vi "Autonomous Independent.vi"   [LabVIEW 2013]
doc: "This VI is called when autonomous begins, and will automatically be terminated when autonomous ends. You can carry out timed or sensor driven robot movement independently without needing to return to the caller."
uses:
  <vilib>/Rock Robotics/WPI/Solenoid/WPI_SolenoidValue.ctl
  Robot Global Data.vi
  <vilib>/Rock Robotics/WPI/RobotDrive/WPI_RobotDriveGetSetRefNum.vi
  <vilib>/Rock Robotics/WPI/Solenoid/WPI_SolenoidSetEnum.vi
  <vilib>/Rock Robotics/WPI/Joystick/WPI_JoystickGetSetRefNum.vi
panel:
  # "Be sure to right-click and choose Data Operations>>Make Current Value default if you want to save the array values with the VI"
types:
  T1 = typedef "WPI_JoystickDevRef.ctl" = cluster{"Device":T2}
  T2 = typedef "WPI_JoystickDeviceEnum.ctl" = enum16{"USB 1", "USB 2", "USB 3", "USB 4", "Kinect 1", "Kinect 2"}
  T3 = cluster{"axis 1 (x)":dbl, "axis 2 (y)":dbl, "axis 3 (throttle)":dbl, "axis 4":dbl, "axis 5":dbl, "axis 6":dbl}
  T4 = typedef "WPI_RobotDriveDevRef.ctl" = cluster{"DevStatus":errorcluster, "Motors[]":T5[], "Square Inputs":bool, "Max Output":dbl, "Isochronous":bool}
  T5 = typedef "WPI_MotorControlDeviceRef.ctl" = cluster{"DeviceStatus":errorcluster, "Type":enum16{"PWM", "CAN"}, "PWM":cluster{"Digital Module":T6, "PWM Channel":T7, "DeadBand":T8}, "CAN":cluster{"Device Number":u8, "Control Mode":T9, "Semaphore":T10, "Max Vout":dbl}, "Invert":bool, "TransformRef":T11, "InvTransformRef":T11}
  T6 = typedef "FPGA_TypedefDigitalModule.ctl" = enum16{"Digital Module 1", "Digital Module 2"}
  T7 = typedef "FPGA_DIOPWMChannel.ctl" = enum8{"PWM 1", "PWM 2", "PWM 3", "PWM 4", "PWM 5", "PWM 6", "PWM 7", "PWM 8", "PWM 9", "PWM 10", "Invalid"}
  T8 = typedef "WPI_PWMDeadband.ctl" = cluster{"Name":string, "maxPositivePwm":i32, "minPositivePwm":i32, "centerPwm":i32, "maxNegativePwm":i32, "minNegativePwm":i32, "angularRange":u16}
  T9 = typedef "WPI_CANJaguar_ControlMode.ctl" = enum8{"Percent VBus", "Current", "Speed", "Position", "Voltage"}
  T10 = typedef "Semaphore RefNum" = refnum<k1>
  T11 = typedef "WPI_PWMTransform_ConPane.ctl" = refnum<vi>
  T12 = typedef "WPI_SolenoidDevRef.ctl" = cluster{"DevStatus":errorcluster, "Solenoid Module":T13, "Forward Solenoid Channel":T14, "Reverse Solenoid Channel":T14}
  T13 = typedef "FPGA_TypedefSolenoidModule.ctl" = enum16{"Solenoid Module 1", "Solenoid Module 2"}
  T14 = typedef "WPI_SolenoidChannel.ctl" = enum8{"Solenoid 1", "Solenoid 2", "Solenoid 3", "Solenoid 4", "Solenoid 5", "Solenoid 6", "Solenoid 7", "Solenoid 8", "Invalid"}
  T15 = typedef "WPI_SolenoidValue.ctl" = enum16{"Off", "On", "Forward", "Reverse"}
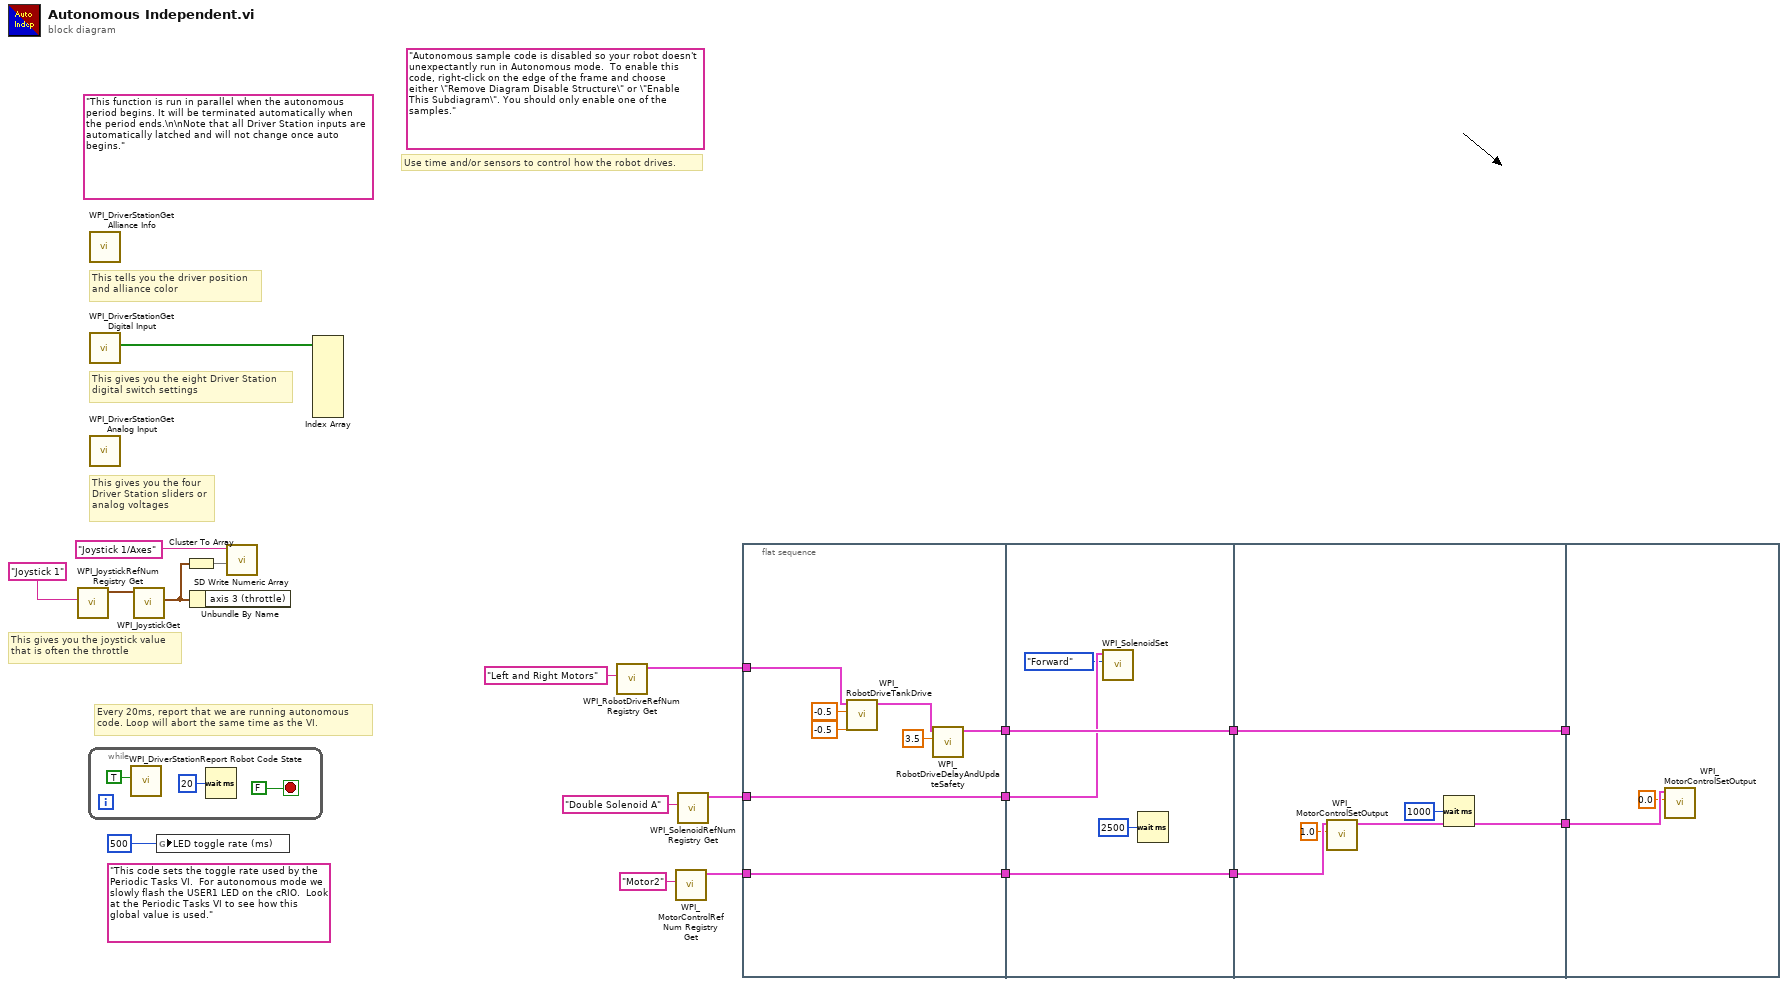
[diagram p0: block diagram]
diagram:
  (unwired) "This code sets the toggle rate used by the Periodic Tasks VI.  For autonomous mode we slowly flash the USER1 LED on the cRIO.  Look at the Periodic Tasks VI to see how this global value is used."
  (unwired) "Autonomous sample code is disabled so your robot doesn't unexpectantly run in Autonomous mode.  To enable this code, right-click on the edge of the frame and choose either \"Remove Diagram Disable Structure\" or \"Enable This Subdiagram\". You should only enable one of the samples."
  (unwired) "This function is run in parallel when the autonomous period begins. It will be terminated automatically when the period ends.\n\nNote that all Driver Station inputs are automatically latched and will not change once auto begins."
  # "This gives you the joystick value\nthat is often the throttle"
  # "Every 20ms, report that we are running autonomous\ncode. Loop will abort the same time as the VI."
  # "Use time and/or sensors to control how the robot drives."
  # "This tells you the driver position\nand alliance color"
  # "This gives you the eight Driver Station\ndigital switch settings"
  # "This gives you the four\nDriver Station sliders or\nanalog voltages"
  n1 = call <vilib>:"WPI_JoystickRefNum Registry Get.vi"("refnum name"="Joystick 1") -> ("JoystickDevRef"=w17:T1)  [unwired: 1 in, 9 out]
  n2 = while {
    stop <- FALSE stop-if-true
    n3 = call <vilib>:"WPI_DriverStationReport Robot Code State.vi"("Autonomous"=TRUE) -> ()  [unwired: 10 in, 1 out]
    n4 = Wait (ms)(milliseconds to wait=u32 20) -> ()  [unwired: 1 out]
  }
  n5 = call <vilib>:"WPI_DriverStationGet Alliance Info.vi"() -> ()  [unwired: 12 out]
  n6 = call <vilib>:"WPI_DriverStationGet Digital Input.vi"() -> ("Driver Station Digital Input (1-8)"=w20:bool[])  [unwired: 11 out]
  n7 = call <vilib>:"WPI_DriverStationGet Analog Input.vi"() -> ()  [unwired: 12 out]
  n8 = call <vilib>:"WPI_JoystickGet.vi"("JoystickDevRef"=w17) -> ("Axes"=w15:T3)  [unwired: 1 in, 5 out]
  n9 = global write "Robot Global Data.vi" "LED toggle rate (ms)"(u32 500 ("LED ms toggle rate")) -> ()
  n10 = Cluster To Array(cluster=w15) -> (array=w16:dbl[])
  n11 = Unbundle By Name(w15) -> ()  [unwired: 1 out]
  n12 = call <vilib>:"SD Write Numeric Array.vi"("Numeric Array"=w16, "Name"="Joystick 1/Axes") -> ()  [unwired: 8 in, 2 out]
  n13 = Index Array(array=w20) -> ()  [unwired: 8 in, 8 out]
  n14 = call <vilib>:"WPI_RobotDriveRefNum Registry Get.vi"("refnum name"="Left and Right Motors") -> ("RobotDriveDevRef"=w12:T4)  [unwired: 9 in, 1 out]
  n15 = call <vilib>:"WPI_MotorControlRefNum Registry Get.vi"("refnum name"="Motor2") -> ("MotorControlDevRef"=w10:T5)  [unwired: 9 in, 1 out]
  n16 = call <vilib>:"WPI_SolenoidRefNum Registry Get.vi"("refnum name"="Double Solenoid A") -> ("SolenoidDevRef"=w2:T12)  [unwired: 9 in, 1 out]
  n17 = flat-sequence {
    tunnel: w12 -> [w27]
    tunnel: [w26] -> w8
    tunnel: [w25] -> w6
    tunnel: w10 -> [w25]
    tunnel: [w24] -> w3
    tunnel: w2 -> [w24]
    tunnel: w8 -> [w36]
    tunnel: [w36] -> w7
    tunnel: w6 -> [w35]
    tunnel: [w35] -> w5
    tunnel: w3 -> [w34]
    tunnel: w7 -> [w41]
    tunnel: w5 -> [w40]
    tunnel: [w41] -> w9
    tunnel: [w37] -> w1
    tunnel: w9 -> [_]
    tunnel: w1 -> [w43]
    frame #0 {
      n18 = call <vilib>:"WPI_RobotDriveTankDrive.vi"("Right axis value"=-0.5, "Left axis value"=-0.5, "RobotDriveDevRef"=w27) -> ("RobotDriveDevRef"=w29:T4)  [unwired: 6 in, 2 out]
      n19 = call <vilib>:"WPI_RobotDriveDelayAndUpdateSafety.vi"("Delay (s)"=3.5, "RobotDriveDevRef"=w29) -> ("RobotDriveDevRef 2"=w26:T4)  [unwired: 8 in, 1 out]
    }
    frame #1 {
      n20 = call-poly <vilib>:"WPI_SolenoidSet.vi"("Value"=WPI_SolenoidValue."Forward", "SolenoidDevRef"=w34) -> ()  [unwired: 8 in, 2 out]
      n21 = Wait (ms)(milliseconds to wait=u32 2500) -> ()  [unwired: 1 out]
    }
    frame #2 {
      n22 = call <vilib>:"WPI_MotorControlSetOutput.vi"("Output"=1.0, "MotorControlDevRef"=w40) -> ("MotorControlDevRef"=w37:T5)  [unwired: 7 in, 2 out]
      n23 = Wait (ms)(milliseconds to wait=u32 1000) -> ()  [unwired: 1 out]
    }
    frame #3 {
      n24 = call <vilib>:"WPI_MotorControlSetOutput.vi"("Output"=0.0, "MotorControlDevRef"=w43) -> ()  [unwired: 7 in, 3 out]
    }
  }
